vi "Get_Values.vi"(0 "reference in":refnum<class "Sig_AO.lvclass">) -> (6 "AO":dbl)   [LabVIEW 2019, in "Sig_AO.lvclass"]
uses:
  Sig_AO.lvclass
  Sig_AO.lvclass/Sig_AO.ctl
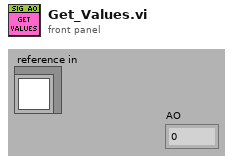
[diagram p1: front panel]
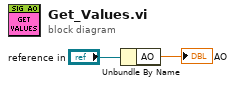
[diagram p0: block diagram]
diagram:
  n1 = Unbundle By Name("reference in") -> ("AO"=→"AO":dbl)
